vi "Mouse Up.vi"(7 "Map Model in":refnum<class "Map Model.lvclass">, 8 "error in (no error)":errorcluster, 10 "Position":T1, 11 "Rectangle Select in":refnum<class "Rectangle Select.lvclass">) -> (0 "error out":errorcluster, 3 "Rectangle Select out":refnum<class "Rectangle Select.lvclass">, 5 "Map Model out":refnum<class "Map Model.lvclass">)   [LabVIEW 2020, in "Map Model.lvlib" / "Rectangle Select.lvclass"]
uses:
  Rectangle Select.lvclass
  E:/Project/Labview-Projects/Completed projects/Map Editor/Models/Map Model/Tools/Tool/Tool.lvclass
  <vilib>/Utility/miscctls.llb/LVPoint32TypeDef.ctl
  Map Model/Map Model.lvclass
  Tool/Tool.lvclass/Tool.ctl
  Map Model/Map Model.lvclass/Map Model.ctl
  Tool/Tool.lvclass
panel:
  # "NOTICE -- YOU MUST LEAVE THIS NOTICE IN PLACE.\n\nCopyright (c) 2017, LIANG LIU Shawn.Liu.cn@gmail.com\nAll rights reserved.\n\nRedistribution and use in source and binary forms, with or without modification, are permitted provided that the following conditions are met:\n-Redistributions of source code must retain the above copyright notice, this list of conditions and the following disclaimer.\n-Redistributions in binary form must reproduce the above copyright notice, this list of conditions and the following disclaimer in the documentation and/or other materials provided with the distribution.\n-Neither the name of the eLp nor the names of its contributors may be used to endorse or promote products derived from this software without specific prior written permission.\n\nTHIS SOFTWARE IS PROVIDED BY THE COPYRIGHT HOLDERS AND CONTRIBUTORS \"AS IS\" AND ANY EXPRESS OR IMPLIED WARRANTIES, INCLUDING, BUT NOT LIMITED TO, THE IMPLIED WARRANTIES OF MERCHANTABILITY AND FITNESS FOR A PARTICULAR PURPOSE ARE DISCLAIMED. IN NO EVENT SHALL THE COPYRIGHT HOLDER OR CONTRIBUTORS BE LIABLE FOR ANY DIRECT, INDIRECT, INCIDENTAL, SPECIAL, EXEMPLARY, OR CONSEQUENTIAL DAMAGES (INCLUDING, BUT NOT LIMITED TO, PROCUREMENT OF SUBSTITUTE GOODS OR SERVICES; LOSS OF USE, DATA, OR PROFITS; OR BUSINESS INTERRUPTION) HOWEVER CAUSED AND ON ANY THEORY OF LIABILITY, WHETHER IN CONTRACT, STRICT LIABILITY, OR TORT (INCLUDING NEGLIGENCE OR OTHERWISE) ARISING IN ANY WAY OUT OF THE USE OF THIS SOFTWARE, EVEN IF ADVISED OF THE POSSIBILITY OF SUCH DAMAGE."
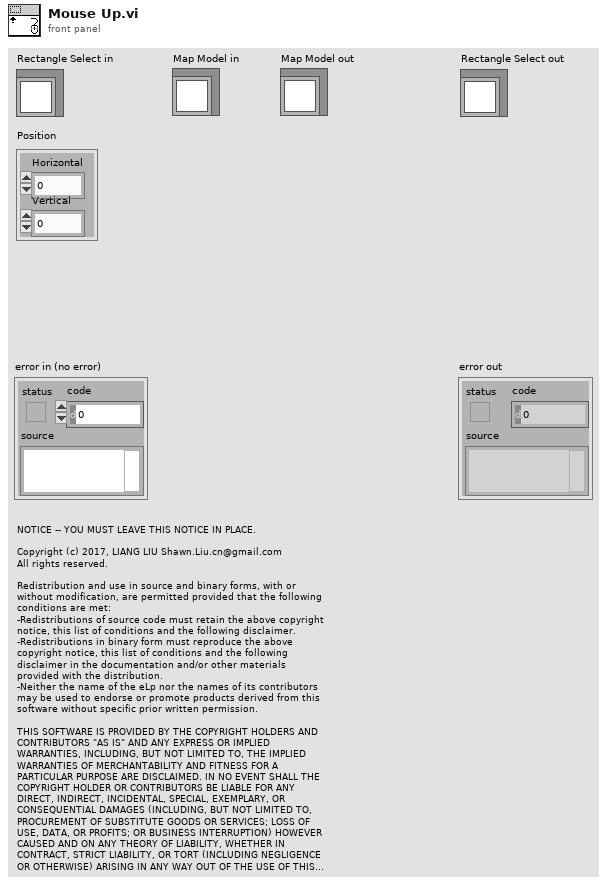
[diagram p1: front panel]
types:
  T1 = typedef "LVPoint32TypeDef.ctl" = cluster{"Horizontal":i32, "Vertical":i32}
  T2 = enum8{"Enabled", "Disabled", "Disabled and Grayed Out"}
  T3 = cluster{"Occupied Color":cluster{"Value":u8, "Color":u32}, "Free Color":cluster{"Value":u8, "Color":u32}, "Unknown Color":cluster{"Value":u8, "Color":u32}}
  T4 = cluster{"left":i16, "top":i16, "right":i16, "bottom":i16}
  T5 = typedef "LVPointTypeDef.ctl" = cluster{"Horizontal":i16, "Vertical":i16}
  T6 = typedef "imagedata.ctl" = cluster{"image type":i32, "image depth":i32, "image":u8[], "mask":u8[], "colors":u32[], "Rectangle":cluster{"left":i16, "top":i16, "right":i16, "bottom":i16}}
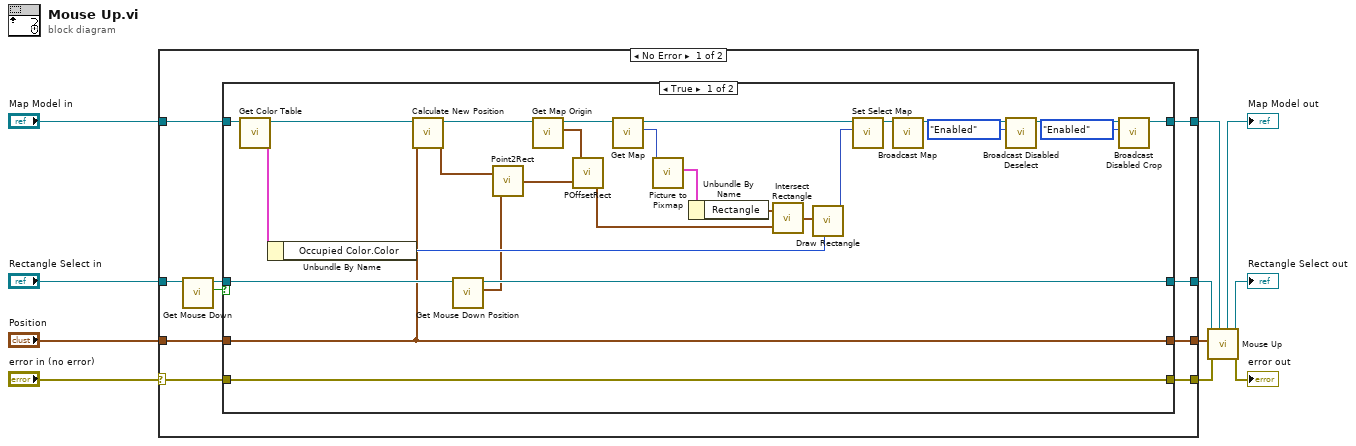
[diagram p0: block diagram]
diagram:
  n1 = case shown="No Error" "error in (no error)" {
    selector: "error in (no error)" -> [w18 w56]
    tunnel: "Map Model in" -> [w21 w55]
    tunnel: "Rectangle Select in" -> [w20 w54]
    tunnel: "Position" -> [w19 w53]
    tunnel: [w17 w53] -> w7
    tunnel: [w16 w55] -> w5
    tunnel: [w15 w54] -> w6
    tunnel: [w12 w56] -> w4
    frame No Error {
      n2 = call "Get Mouse Down.vi"("Tool in"=w20) -> ("Mouse Down"=w13:bool, "Tool out"=w14:refnum<class "Rectangle Select.lvclass">)  [unwired: 9 in]
      n3 = case shown="True" w13 {
        tunnel: w14 -> [w48 w52]
        tunnel: w21 -> [w47 w50]
        tunnel: [w23 w50] -> w16
        tunnel: [w46 w52] -> w15
        tunnel: w19 -> [w41 w49]
        tunnel: [w41 w49] -> w17
        tunnel: w18 -> [w42 w51]
        tunnel: [w42 w51] -> w12
        frame True {
          n4 = call "Get Color Table.vi"("Map Model in"=w47) -> ("Color Table"=w44:T3, "Map Model out"=w45:refnum<class "Map Model.lvclass">)  [unwired: 9 in]
          n5 = Unbundle By Name(w44) -> ("Occupied Color.Color"=w43:u32)
          n6 = call "Calculate New Position.vi"("Position in"=w41, "Map Model in"=w45) -> ("Position out"=w39:T1, "Map Model out"=w34:refnum<class "Map Model.lvclass">)  [unwired: 8 in]
          n7 = call "Get Mouse Down Position.vi"("Tool in"=w48) -> ("Mouse Down Position"=w40:T1, "Tool out"=w46:refnum<class "Rectangle Select.lvclass">)  [unwired: 9 in]
          n8 = call <vilib>:"Point2Rect.vi"("point b"=w40, "point a"=w39) -> ("rect"=w32:T4)
          n9 = call "Get Map Origin.vi"("Map Model in"=w34) -> ("Map Origin"=w28:T5, "Map Model out"=w33:refnum<class "Map Model.lvclass">)  [unwired: 9 in]
          n10 = call <vilib>:"POffsetRect.vi"("rect"=w32, "point"=w28) -> ("offset rect"=w31:T4)
          n11 = call "Get Map.vi"("Map Model in"=w33) -> ("Map"=w38:picture, "Map Model out"=w29:refnum<class "Map Model.lvclass">)  [unwired: 9 in]
          n12 = call <vilib>:"Picture to Pixmap.vi"("picture"=w38) -> ("image data"=w26:T6)  [unwired: 9 in, 1 out]
          n13 = Unbundle By Name(w26) -> ("Rectangle"=w37:T4)
          n14 = call "Intersect Rectangle.vi"("Rectangle B"=w31, "Rectangle A"=w37) -> ("Intersect Rectangle"=w30:T4)
          n15 = call <vilib>:"Draw Rectangle.vi"("rect"=w30, "color(black)"=w43) -> ("new picture"=w27:picture)  [unwired: 7 in]
          n16 = call "Set Select Map.vi"("Select Map"=w27, "Map Model in"=w29) -> ("Map Model out"=w36:refnum<class "Map Model.lvclass">)  [unwired: 9 in]
          n17 = call "Broadcast Map.vi"("Map Model in"=w36) -> ("Map Model out"=w35:refnum<class "Map Model.lvclass">)  [unwired: 9 in, 1 out]
          n18 = call "Broadcast Disabled Deselect.vi"("Disabled Deselect"=T2."Enabled", "Map Model in"=w35) -> ("Map Model out"=w25:refnum<class "Map Model.lvclass">)  [unwired: 8 in, 1 out]
          n19 = call "Broadcast Disabled Crop.vi"("Disabled Crop"=T2."Enabled", "Map Model in"=w25) -> ("Map Model out"=w23:refnum<class "Map Model.lvclass">)  [unwired: 8 in, 1 out]
        }
        frame False {
        }
      }
    }
    frame Error {
    }
  }
  n20 = call-parent "Mouse Up.vi"("Map Model in"=w5, "error in (no error)"=w4, "Position"=w7, "Tool in"=w6) -> ("error out"=→"error out":errorcluster, "Tool out"=→"Rectangle Select out":refnum<class "Rectangle Select.lvclass">, "Map Model out"=→"Map Model out":refnum<class "Map Model.lvclass">)  [unwired: 5 in]
